vi "Build Major Frame.vi"(8 "error in (no error)":errorcluster, 11 "Bus Controller XML Node":refnum<k20>) -> (0 "error out":errorcluster, 3 "Major Frame out":refnum<class "Major Frame.lvclass">)   [LabVIEW 2016]
doc: "Reads the Bus Controller node to produce an entire Major Frame schedule. The Major Frame, Minor Frames, and Messages all get constructed here."
uses:
  Frames & Messages/Major Frame/Major Frame.lvclass
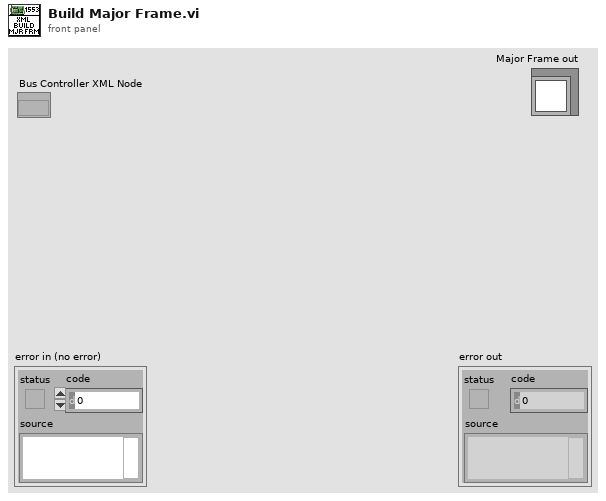
[diagram p1: front panel]
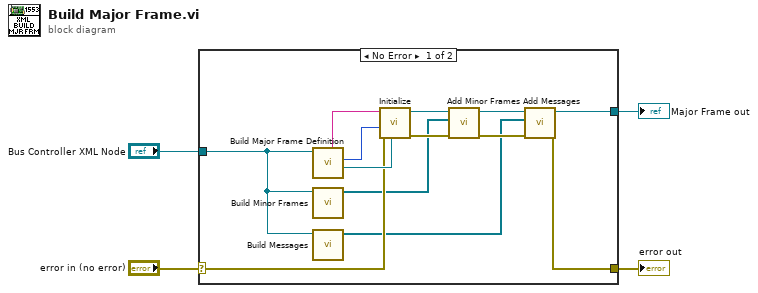
[diagram p0: block diagram]
diagram:
  n1 = case shown="No Error" "error in (no error)" {
    selector: "error in (no error)" -> [w9 w18]
    tunnel: [w8 w18] -> w3
    tunnel: "Bus Controller XML Node" -> [w7 _]
    tunnel: [w12 _] -> w1
    frame No Error {
      n2 = call "Build Major Frame Definition.vi"("Bus Controller XML Node"=w7) -> ("Major Schedule"=w16:refnum<queue>, "Minor Frame Rate"=w15:u16, "Major Frame ID"=w17:string)  [unwired: 7 in, 1 out]
      n3 = call "Build Minor Frames.vi"("Bus Controller XML Node"=w7) -> ("Minor Frames"=w6:refnum<class "Minor Frame.lvclass">[])  [unwired: 9 in, 1 out]
      n4 = call "Build Messages.vi"("Bus Controller XML Node"=w7) -> ("Messages"=w5:refnum<class "Message.lvclass">[])  [unwired: 9 in, 1 out]
      n5 = call "Initialize.vi"("Schedule"=w16, "error in (no error)"=w9, "Minor Frame Time (100 us)"=w15, "ID"=w17) -> ("error out"=w11:errorcluster, "Major Frame out"=w13:refnum<class "Major Frame.lvclass">)  [unwired: 6 in]
      n6 = call-dynamic "Add Minor Frames.vi"("error in (no error)"=w11, "Minor Frames"=w6, "Major Frame in"=w13) -> ("error out"=w10:errorcluster, "Major Frame out"=w14:refnum<class "Major Frame.lvclass">)  [unwired: 7 in]
      n7 = call-dynamic "Add Messages.vi"("error in (no error)"=w10, "Messages"=w5, "Major Frame in"=w14) -> ("error out"=w8:errorcluster, "Major Frame out"=w12:refnum<class "Major Frame.lvclass">)  [unwired: 7 in]
    }
    frame Error {
    }
  }
  "error out" <- w3
  "Major Frame out" <- w1
